vi "数组拆分.vi"(10 "拆分间隔":i32=300, 11 "all rows":dbl[][](array[numeric])) -> (3 "数组":cluster{dbl[][]}[](array[cluster]))   [LabVIEW 2016]
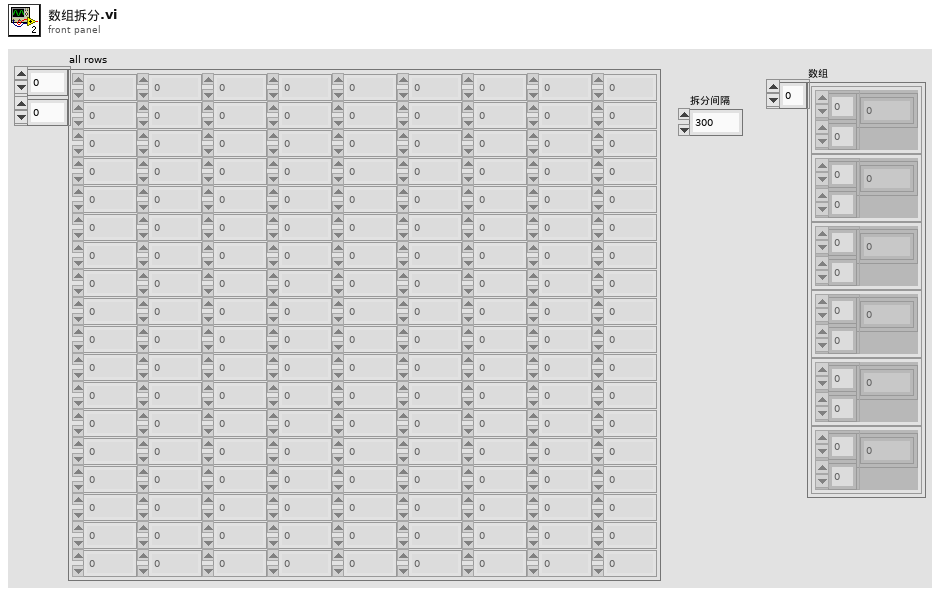
[diagram p1: front panel]
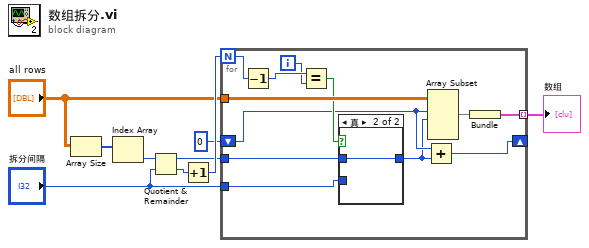
[diagram p0: block diagram]
diagram:
  n1 = Array Size(array="all rows") -> (size(s)=w9:i32[])
  n2 = Index Array(array=w9) -> (element=w8:i32)  [unwired: 1 in]
  n3 = Quotient & Remainder(x=w8, y="拆分间隔") -> (x-y*floor(x/y)=w4:i32, floor(x/y)=w7:i32)
  n4 = Increment(x=w7) -> (x+1=w6:i32)
  n5 = for {
    N: w6 -> [w20]
    tunnel: "all rows" -> [w21]
    tunnel: w4 -> [w16]
    tunnel: "拆分间隔" -> [w15]
    shift-right: [w12] -> _
    shift-left: 0 ("索引") -> [w14]
    tunnel: [w10] -> w1 mode=indexing
    i -> [w18]
    n6 = Decrement(x=w20) -> (x-1=w19:i32)
    n7 = Equal?(x=w19, y=w18) -> (x = y?=w17:bool)
    n8 = case shown="真" w17 {
      tunnel: w16 -> [_ w23]
      tunnel: [w22 w23] -> w13
      tunnel: w15 -> [w22 _]
      frame False {
      }
      frame True {
      }
    }
    n9 = Add(x=w14, y=w13) -> (x+y=w12:i32)
    n10 = Array Subset(array=w21, index (row)=w14, length (row)=w13) -> (w11:dbl[][])  [unwired: 2 in]
    n11 = Bundle(w11) -> (w10:cluster{dbl[][]})  [unwired: 1 in]
  }
  "数组" <- w1
